vi "Revision Query.vi"(8 "error in (no error)":errorcluster, 11 "VISA resource name":refnum<visa-resource-name>) -> (0 "error out":errorcluster, 1 "Instr Firmware Revision":string, 2 "Instr Driver Revision":string, 3 "VISA resource name out":refnum<visa-resource-name>)   [LabVIEW 2020, in "Yokogawa GX Series.lvlib"]
doc: "Queries the current instrument firmware revision and instrument driver revision.\n\nFor detailed driver information including modification history, refer to the <B> Yokogawa GX Series Readme.html </B> file."
uses:
  <instrlib>/Yokogawa GX Series/Yokogawa GX Series.lvlib
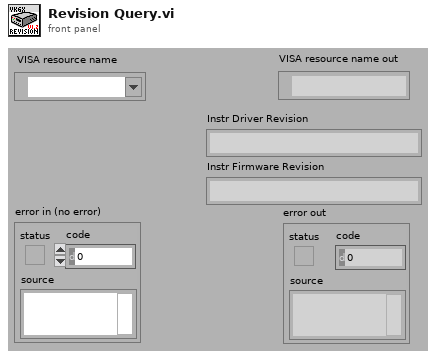
[diagram p1: front panel]
types:
  T1 = enum32{"invalid app kind", "Development System", "Run Time System", "Student Edition", "Embedded LabVIEW", "Evaluation", "Custom"}
  T2 = cluster{"Major":u16, "Minor":u16, "Fix":u16, "Build":u16}
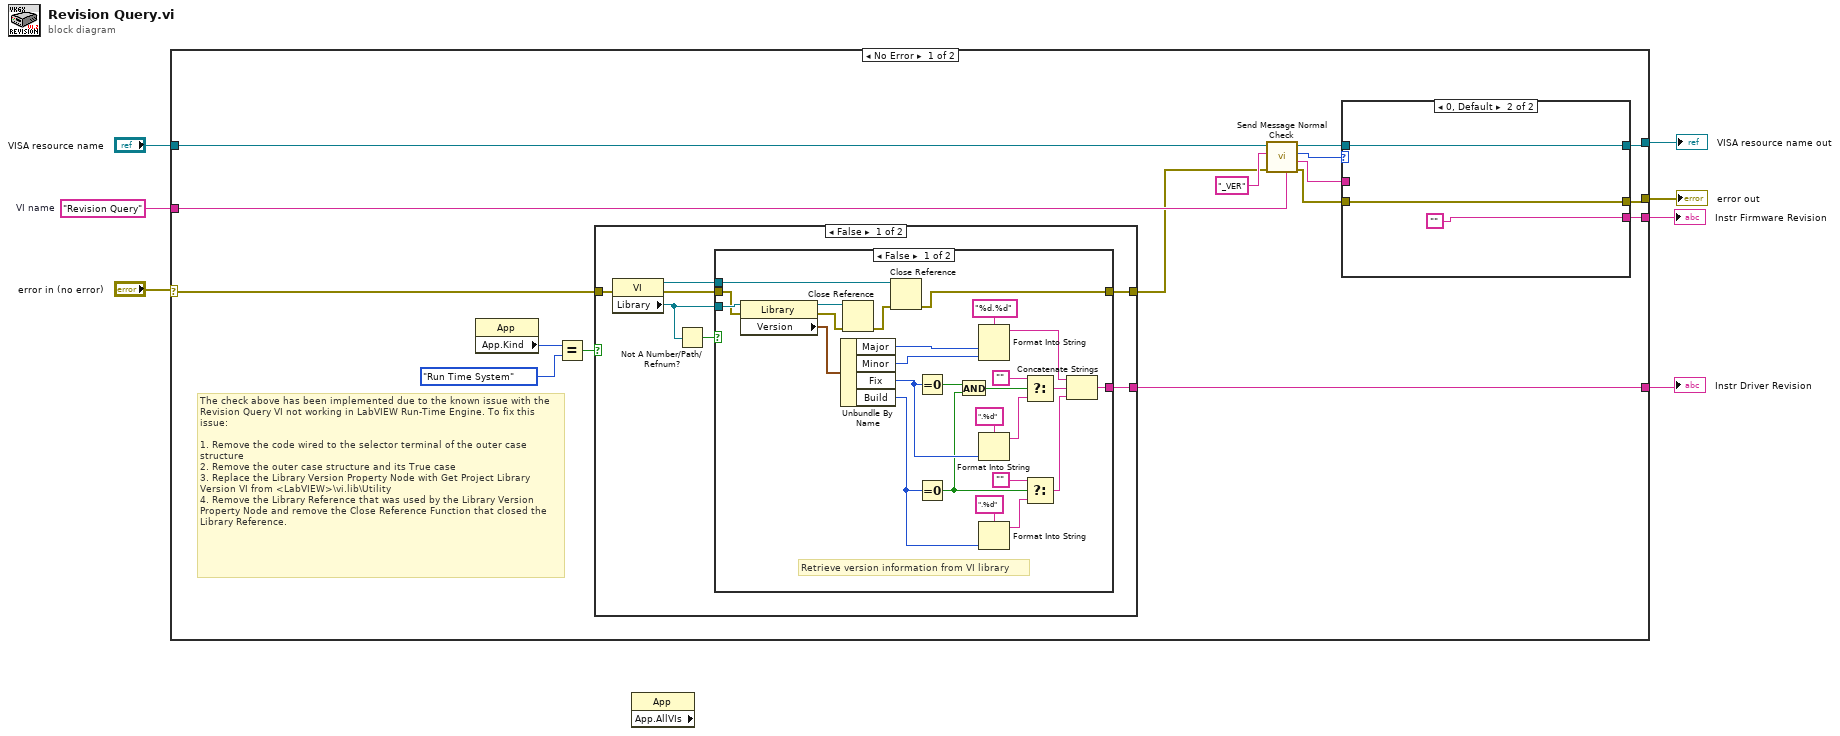
[diagram p0: block diagram]
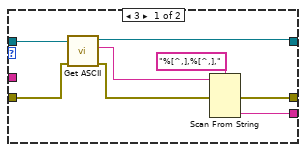
[diagram p2: hidden frame]
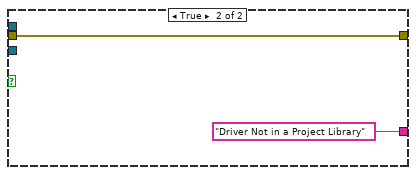
[diagram p3: hidden frame]
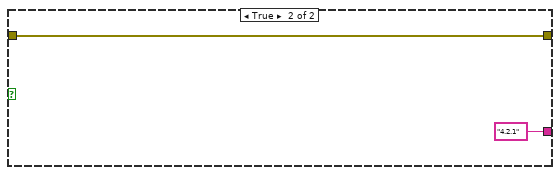
[diagram p4: hidden frame]
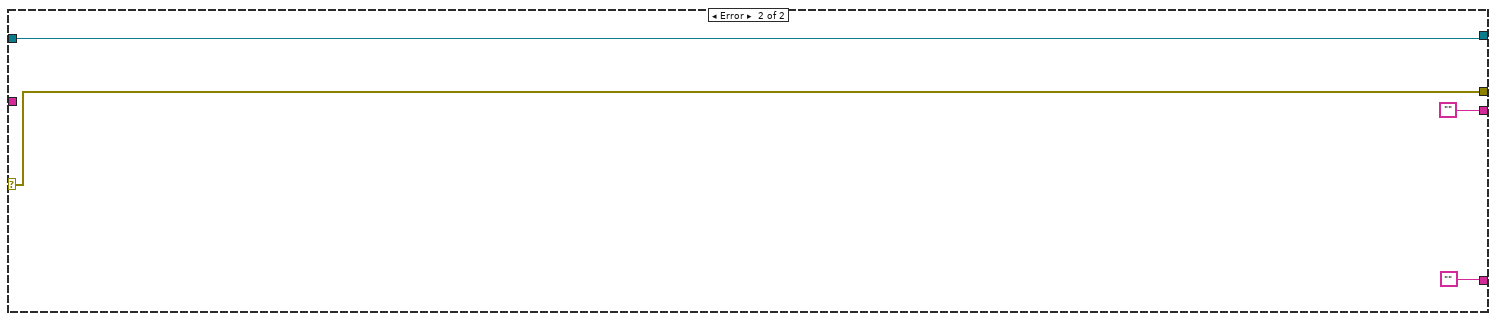
[diagram p5: hidden frame]
diagram:
  w7 = "Revision Query"  # VI name
  n1 = case shown="No Error" "error in (no error)" {
    selector: "error in (no error)" -> [w8 w74]
    tunnel: w7 -> [w23 _]
    tunnel: [w22 w74] -> w6
    tunnel: [w15 ""] -> w5
    tunnel: [w12 w75] -> w4
    tunnel: "VISA resource name" -> [w10 w75]
    tunnel: [w9 ""] -> w2
    frame No Error {
      # "The check above has been implemented due to the known issue with the Revision Query VI not working in LabVIEW Run-Time Engine. To fix this issue:\n\n1. Remove the code wired to the selector terminal of the outer case structure\n2. Remove the outer case structure and its True case\n3. Replace the Library Version Property Node with Get Project Library Version VI from <LabVIEW>\\vi.lib\\Utility\n4. Remove the Library Reference that was used by the Library Version Property Node and remove the Close Reference Function that closed the Library Reference."
      n2 = property class="App"() -> ("App.Kind"=w20:T1)  [unwired: 2 in, 2 out]
      n3 = Equal?(x=w20, y=T1."Run Time System" ("Application:Kind")) -> (x = y?=w21:bool)
      n4 = case shown="False" w21 {
        tunnel: [w40 "4.2.1"] -> w9
        tunnel: w8 -> [w38 w70]
        tunnel: [w39 w70] -> w16
        frame False {
          n5 = property class="VI"(error in=w38) -> (reference out=w36:refnum<vi>, error out=w35:errorcluster, "Library"=w37:refnum<vi>)  [unwired: 1 in]
          n6 = Not A Number/Path/Refnum?(number/path/refnum=w37) -> (NaN/Path/Refnum?=w41:bool)
          n7 = case shown="False" w41 {
            tunnel: [w47 w68] -> w39
            tunnel: [w46 "Driver Not in a Project Library"] -> w40
            tunnel: w37 -> [w44 _]
            tunnel: w36 -> [w43 _]
            tunnel: w35 -> [w42 w68]
            frame False {
              # "Retrieve version information from VI library"
              n8 = property class="Library"(reference=w44, error in=w42) -> (reference out=w66:refnum<vi>, error out=w67:errorcluster, "Version"=w64:T2)
              n9 = Unbundle By Name(w64) -> ("Major"=w54:u16, "Minor"=w53:u16, "Fix"=w51:u16, "Build"=w52:u16)
              n10 = Close Reference(reference=w66, error in (no error)=w67) -> (error out=w65:errorcluster)
              n11 = Close Reference(reference=w43, error in (no error)=w65) -> (error out=w47:errorcluster)
              n12 = Equal To 0?(x=w51) -> (x = 0?=w50:bool)
              n13 = Equal To 0?(x=w52) -> (x = 0?=w49:bool)
              n14 = And(x=w50, y=w49) -> (x .and. y?=w48:bool)
              n15 = Format Into String(format string="%d.%d", w54, w53) -> (resulting string=w60:string)  [unwired: 2 in, 1 out]
              n16 = Format Into String(format string=".%d", w51) -> (resulting string=w45:string)  [unwired: 2 in, 1 out]
              n17 = Format Into String(format string=".%d", w52) -> (resulting string=w58:string)  [unwired: 2 in, 1 out]
              n18 = Select(t="", s=w48, f=w45) -> (s? t:f=w59:string)
              n19 = Select(t="", s=w49, f=w58) -> (s? t:f=w55:string)
              n20 = Concatenate Strings(w60, w59, w55) -> (w46:string)
            }
            frame True {
            }
          }
        }
        frame True {
        }
      }
      n21 = call <instrlib>:"Send Message Normal Check.vi"("Source (\"\")"=w23, "error in (no error)"=w16, "Send Message (\"\")"="_VER" ("書き込みバッファ"), "VISA resource name"=w10) -> ("error out"=w17:errorcluster, "Read Buffer"=w11:string, "Response Type"=w14:i32, "VISA resource name out"=w13:refnum<visa-resource-name>)  [unwired: 2 in, 2 out]
      n22 = case shown="0, Default" w14 {
        tunnel: [w31 w33] -> w22
        tunnel: w17 -> [w26 w33]
        tunnel: [w29 ""] -> w15
        tunnel: w13 -> [w28 w34]
        tunnel: [w27 w34] -> w12
        tunnel: w11 -> [_ _]
        frame 3 {
          n23 = call <instrlib>:"Get ASCII.vi"("error in (no error)"=w26, "VISA resource name"=w28) -> ("error out"=w25:errorcluster, "ASCII Data"=w24:string, "VISA resource name out"=w27:refnum<visa-resource-name>)  [unwired: 7 in]
          n24 = Scan From String(format string="%[^,],%[^,],", input string=w24, error in=w25) -> (error out=w31:errorcluster, output 2=w29:string)  [unwired: 1 in, 5 out]
        }
        frame 0, Default {
        }
      }
    }
    frame Error {
    }
  }
  "VISA resource name out" <- w4
  "error out" <- w6
  "Instr Firmware Revision" <- w5
  "Instr Driver Revision" <- w2
  n25 = property class="App" props=["App.AllVIs"]() -> ()  [unwired: 2 in, 3 out]
